vi "Lookup Value.vi"(8 "error in (no error)":errorcluster, 10 "Name":string, 11 "Session in":refnum<class "Session.lvclass">) -> (0 "error out":errorcluster, 1 "Not Found?":bool, 2 "Value":string, 3 "Session out":refnum<class "Session.lvclass">)   [LabVIEW 2020, in "HTTP Server.lvlib" / "Session.lvclass"]
uses:
  Session.lvclass
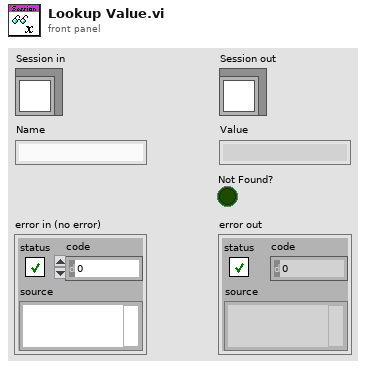
[diagram p1: front panel]
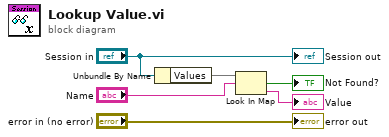
[diagram p0: block diagram]
diagram:
  n1 = Unbundle By Name("Session in") -> ("Values"=w4:map{string, string})
  n2 = Look In Map(map=w4, key="Name") -> (key not found?=→"Not Found?":bool, value=→"Value":string)  [unwired: 1 in]
  "error out" <- "error in (no error)"
  "Session out" <- "Session in"
